vi "Get Data Bit.vi"(8 "error in (no error)":errorcluster caption="entrée d'erreur (pas d'erreur)", 11 "Class Instrument UART en entrée":refnum<class "Class Instrument UART.lvclass">) -> (0 "error out":errorcluster caption="sortie d'erreur", 2 "Data Bit":u16, 3 "Class Instrument UART en sortie":refnum<class "Class Instrument UART.lvclass">)   [LabVIEW 2020, in "Library Instrument & Equipement.lvlib" / "Library Instruments.lvlib" / "Class Instrument UART.lvclass"]
uses:
  Class Instrument UART.lvclass
  Class Instrument UART.lvclass/Class Instrument UART.ctl
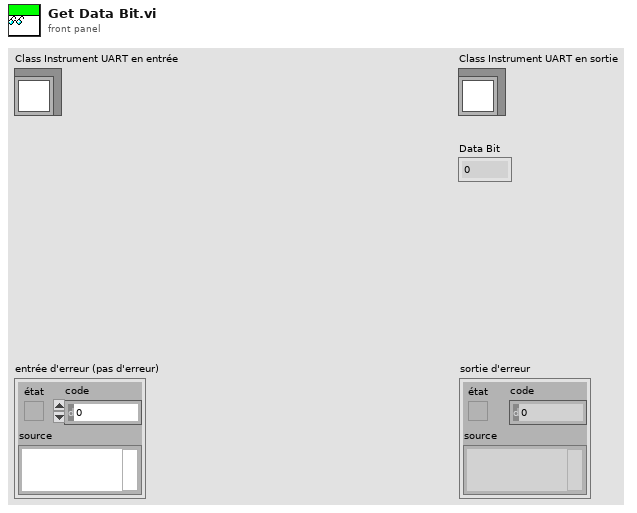
[diagram p1: front panel]
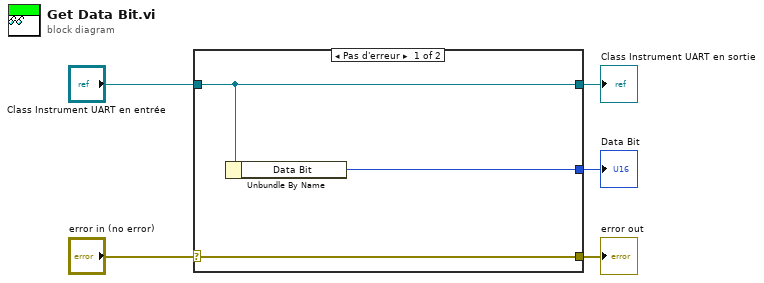
[diagram p0: block diagram]
diagram:
  n1 = case shown="Pas d'erreur" "error in (no error)" {
    selector: "error in (no error)" -> [w8 w9]
    tunnel: [w8 w9] -> w4
    tunnel: [w7 w10] -> w2
    tunnel: "Class Instrument UART en entrée" -> [w7 w10]
    tunnel: [w6 _] -> w1
    frame No Error {
      n2 = Unbundle By Name(w7) -> ("Data Bit"=w6:u16)
    }
    frame Error {
    }
  }
  "error out" <- w4
  "Class Instrument UART en sortie" <- w2
  "Data Bit" <- w1
